vi "GetDrawNumberFromFile.vi"() -> (0 "before substring - Result":string)   [LabVIEW 2023]
uses:
  <vilib>/Utility/file.llb/Read Delimited Spreadsheet (string).vi
panel:
  out "before substring - Result 2":string
  out "spreadsheet string 2":string
  out "subarray 2":string[](array[string])
  out "all rows 2":string[][](array[string])
  out "spreadsheet string":string
  out "subarray":string[](array[string])
  out "all rows":string[][](array[string])
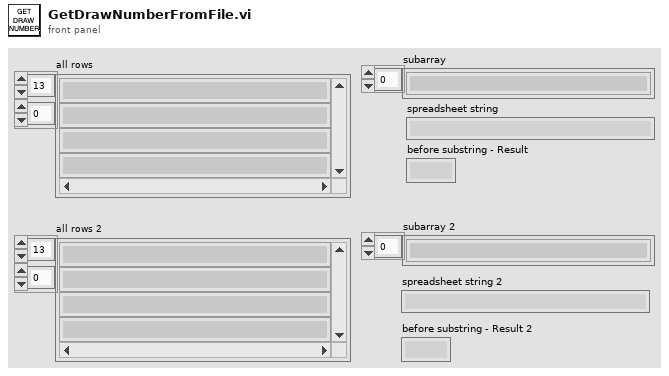
[diagram p1: front panel]
types:
  T1 = enum16{"txtFile to Array", "Get last row", "Array to String", "Pattern", "Stop"}
  T2 = enum16{"txtFile to Array", "Get last row", "Array to String", "Pattern"}
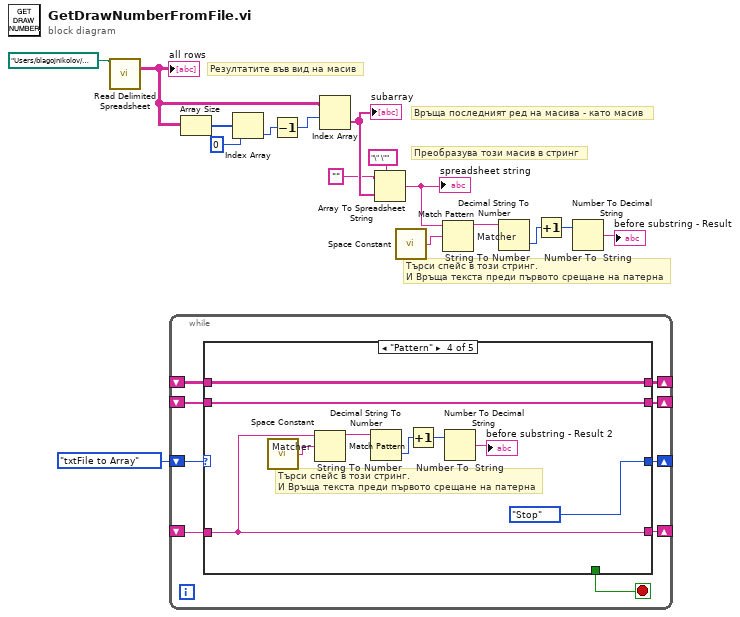
[diagram p0: block diagram]
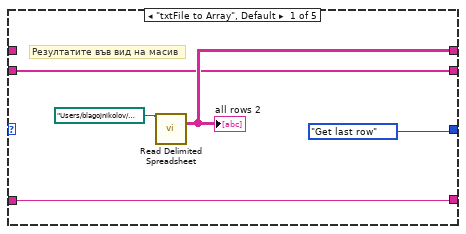
[diagram p2: hidden frame]
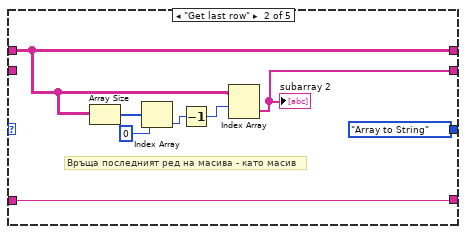
[diagram p3: hidden frame]
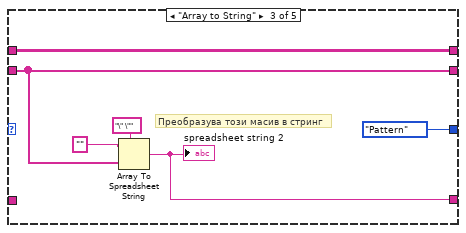
[diagram p4: hidden frame]
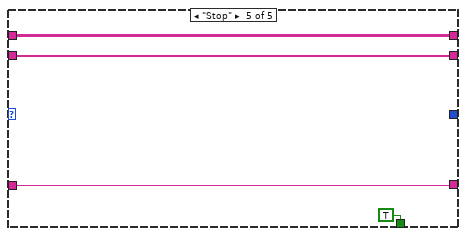
[diagram p5: hidden frame]
diagram:
  # "Търси спейс в този стринг.\nИ Връща текста преди първото срещане на патерна"
  # "Преобразува този масив в стринг"
  # "Връща последният ред на масива - като масив"
  # "Резултатите във вид на масив"
  n1 = call-poly <vilib>:"Read Delimited Spreadsheet.vi"("file path (dialog if empty)"=path "/Users/blagojnikolov/Desktop/@tmp/fromSite.txt") -> ("all rows"=w13:string[][])  [unwired: 9 in, 5 out]
  "all rows" <- w13
  n2 = while {
    shift-right: [w23] -> _
    shift-left: _ -> [w22]
    shift-right: [w25] -> _
    shift-left: T1."txtFile to Array" -> [w24]
    shift-right: [w21] -> _
    shift-left: _ -> [w20]
    shift-right: [w19] -> _
    shift-left: _ -> [w18]
    stop <- w17 stop-if-true
    n3 = case shown="\"Pattern\"" w24 {
      tunnel: [T2."Get last row" T2."Array to String" T2."Pattern" T1."Stop" _] -> w25
      tunnel: [w29 w33 w42 w48 w57] -> w23
      tunnel: w22 -> [_ w33 w42 w48 w57]
      tunnel: [w26 w32 w39 w47 w56] -> w21
      tunnel: w20 -> [w26 _ w39 w47 w56]
      tunnel: [w27 w31 w40 w45 w55] -> w19
      tunnel: w18 -> [w27 w31 _ w45 w55]
      tunnel: [_ _ _ _ TRUE] -> w17
      frame "txtFile to Array", Default {
        # "Резултатите във вид на масив"
        n4 = call-poly <vilib>:"Read Delimited Spreadsheet.vi"("file path (dialog if empty)"=path "/Users/blagojnikolov/Desktop/@tmp/fromSite.txt") -> ("all rows"=w29:string[][])  [unwired: 9 in, 5 out]
        "all rows 2" <- w29
      }
      frame "Get last row" {
        # "Връща последният ред на масива - като масив"
        n5 = Array Size(array=w33) -> (size(s)=w37:i32[])
        n6 = Index Array(array=w37, index=0) -> (element=w35:i32)
        n7 = Decrement(x=w35) -> (x-1=w34:i32)
        n8 = Index Array(array=w33, index (row)=w34) -> (element=w32:string[])  [unwired: 1 in]
        "subarray 2" <- w32
      }
      frame "Array to String" {
        # "Преобразува този масив в стринг"
        n9 = Array To Spreadsheet String(delimiter (Tab)="\" \"", array=w39, 3:"" ("format string")) -> (spreadsheet string=w40:string)
        "spreadsheet string 2" <- w40
      }
      frame "Pattern" {
        # "Търси спейс в този стринг.\nИ Връща текста преди първото срещане на патерна"
        n10 = call <vilib>:"Space Constant.vi"() -> ("String"=w53:string)
        n11 = Match Pattern "Matcher"(string=w45, regular expression=w53) -> (before substring=w52:string)  [unwired: 1 in, 3 out]
        n12 = Decimal String To Number "String To Number"(string=w52) -> (number=w49:i32)  [unwired: 2 in, 1 out]
        n13 = Increment(x=w49) -> (x+1=w51:i32)
        n14 = Number To Decimal String "Number To  String"(number=w51) -> (decimal integer string=→"before substring - Result 2":string)  [unwired: 1 in]
      }
      frame "Stop" {
      }
    }
  }
  n15 = Array Size(array=w13) -> (size(s)=w15:i32[])
  n16 = Index Array(array=w15, index=0) -> (element=w12:i32)
  n17 = Decrement(x=w12) -> (x-1=w11:i32)
  n18 = Index Array(array=w13, index (row)=w11) -> (element=w10:string[])  [unwired: 1 in]
  "subarray" <- w10
  n19 = Array To Spreadsheet String(delimiter (Tab)="\" \"", array=w10, 3:"" ("format string")) -> (spreadsheet string=w7:string)
  "spreadsheet string" <- w7
  n20 = call <vilib>:"Space Constant.vi"() -> ("String"=w6:string)
  n21 = Match Pattern "Matcher"(string=w7, regular expression=w6) -> (before substring=w5:string)  [unwired: 1 in, 3 out]
  n22 = Decimal String To Number "String To Number"(string=w5) -> (number=w2:i32)  [unwired: 2 in, 1 out]
  n23 = Increment(x=w2) -> (x+1=w4:i32)
  n24 = Number To Decimal String "Number To  String"(number=w4) -> (decimal integer string=→"before substring - Result":string)  [unwired: 1 in]
